vi "rx metadata error code.vi"(8 "error in (no error)":errorcluster, 10 "error_code_out":u32(ring) items=["UHD_RX_METADATA_ERROR_CODE_NONE"=0, "UHD_RX_METADATA_ERROR_CODE_TIMEOUT"=1, "UHD_RX_METADATA_ERROR_CODE_LATE_COMMAND"=2, "UHD_RX_METADATA_ERROR_CODE_BROKEN_CHAIN"=4, "UHD_RX_METADATA_ERROR_CODE_OVERFLOW"=8, "UHD_RX_METADATA_ERROR_CODE_ALIGNMENT"=12, "UHD_RX_METADATA_ERROR_CODE_BAD_PACKET"=15], 11 "h":u64) -> (0 "error out":errorcluster, 1 "function return":u32(ring), 2 "error_code_out out":u32(ring) items=["UHD_RX_METADATA_ERROR_CODE_NONE"=0, "UHD_RX_METADATA_ERROR_CODE_TIMEOUT"=1, "UHD_RX_METADATA_ERROR_CODE_LATE_COMMAND"=2, "UHD_RX_METADATA_ERROR_CODE_BROKEN_CHAIN"=4, "UHD_RX_METADATA_ERROR_CODE_OVERFLOW"=8, "UHD_RX_METADATA_ERROR_CODE_ALIGNMENT"=12, "UHD_RX_METADATA_ERROR_CODE_BAD_PACKET"=15], 3 "h out":u64)   [LabVIEW 2023, in "uhd.lvlib"]
doc: "UHD_API uhd_error uhd_rx_metadata_error_code(\n uhd_rx_metadata_handle h, uhd_rx_metadata_error_code_t* error_code_out);"
uses:
  <userlib>/uhd/uhd.lvlib
  <userlib>/uhd/uhd.dll
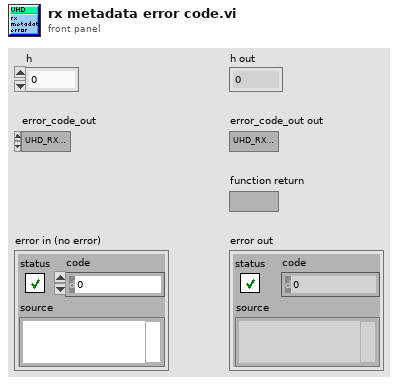
[diagram p1: front panel]
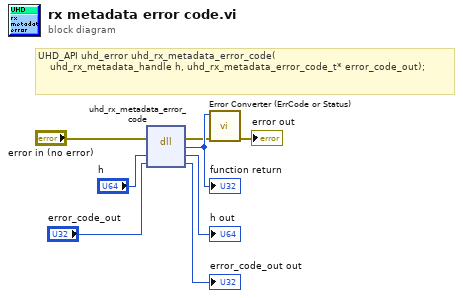
[diagram p0: block diagram]
diagram:
  # "UHD_API uhd_error uhd_rx_metadata_error_code(\n    uhd_rx_metadata_handle h, uhd_rx_metadata_error_code_t* error_code_out);"
  n1 = dll-call lib="C:/Program Files/National Instruments/LabVIEW 2023/user.lib/uhd/uhd.*" fn="uhd_rx_metadata_error_code"(error in="error in (no error)", "h"="h", "error_code_out"="error_code_out") -> (error out=w2:errorcluster, w8:u32, "h"=→"h out":u64, "error_code_out"=→"error_code_out out":u32)  [unwired: 2 in, 1 out]
  "function return" <- w8
  n2 = call <userlib>:"Error Converter (ErrCode or Status).vi"("error in (no error)"=w2, "error code"=w8) -> ("error out"=→"error out":errorcluster)  [unwired: 9 in]
